vi "Get Schedule Shift Aray.vi"(11 "Refnum in":T1) -> (3 "Array":u32[](array[numeric]))   [LabVIEW 2018]
uses:
  <vilib>/Utility/config.llb/Config Data RefNum.ctl
  <vilib>/Utility/config.llb/Read Key (U32).vi
  <vilib>/Utility/config.llb/NI_LVConfig.lvlib
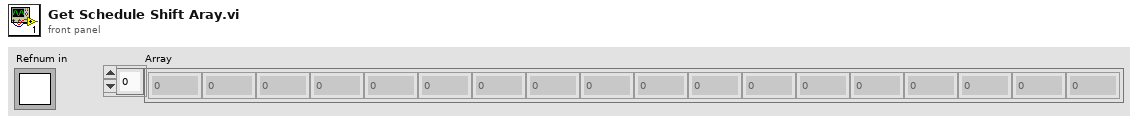
[diagram p1: front panel]
types:
  T1 = typedef "NI_LVConfig.lvlib/Config Data RefNum.ctl" = refnum<k1>
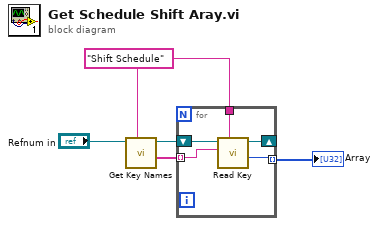
[diagram p0: block diagram]
diagram:
  w3 = "Shift Schedule" ("Shift")
  n1 = call <vilib>:"Get Key Names.vi"("section"=w3, "refnum"="Refnum in") -> ("key names"=w4:string[], "refnum out"=w1:T1)  [unwired: 6 in, 2 out]
  n2 = for {
    tunnel: w3 -> [w10]
    tunnel: [w8] -> w5 mode=indexing
    shift-right: [w7] -> _
    shift-left: w1 -> [w9]
    tunnel: w4 -> [w6] mode=indexing
    n3 = call-poly <vilib>:"Read Key.vi"("section"=w10, "key"=w6, "refnum"=w9) -> ("value"=w8:u32, "refnum out"=w7:T1)  [unwired: 5 in, 2 out]
  }
  "Array" <- w5
